vi "Read Trace.vi"(6 "time_bucket":T1(ring), 7 "max points (-1 = all)":i32=-1 min=-1, 8 "error in (no error)":errorcluster, 9 "time interval":T2, 10 "PG path":string, 11 "Data.PGQL in":refnum<class "LV-Data.PGSQL.lvclass">) -> (0 "error out":errorcluster, 1 "Column (units)":string, 2 "Trace":cluster{timestamp[], dbl[]}, 3 "Data.PGSQL out":refnum<class "LV-Data.PGSQL.lvclass">, 5 "SQL string":string)   [LabVIEW 2019, in "LV-Data.PGSQL.lvclass"]
uses:
  LV-Data.PGSQL.lvclass
  Typedefs/Errors--enum.ctl
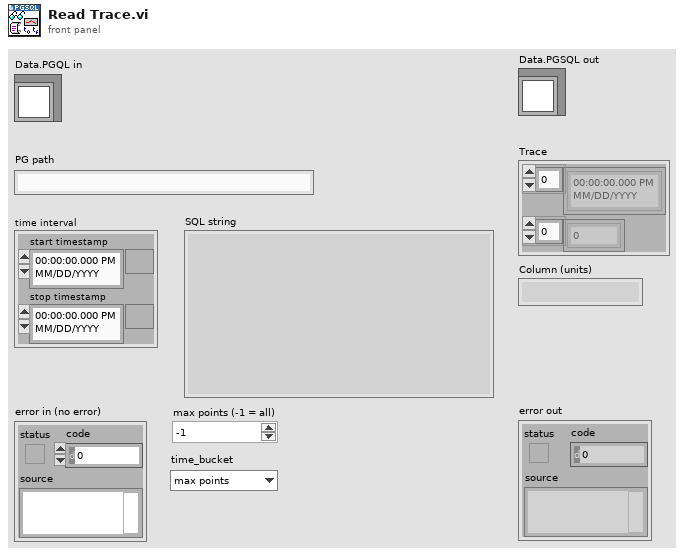
[diagram p1: front panel]
types:
  T1 = enum16{"max points", "1 second", "5 seconds", "10 seconds", "30 seconds", "1 minute", "5 minutes", "10 minutes", "30 minutes", "1 hour", "5 hours", "10 hours", "30 hours"}
  T2 = cluster{"start timestamp":timestamp, "stop timestamp":timestamp}
  T3 = typedef "LV-Data.PGSQL.lvclass/Time.Datatype--enum.ctl" = enum16{"timestamp without time zone", "timestamp with time zone"}
  T4 = typedef "LV-Data.PGSQL.lvclass/Errors--enum.ctl" = enum16{"0: None", "5005: Path Type Not Supported", "5006: Number of Variables", "5007: Number of data points", "5008: Cannot write two data points", "5030: Start and End Times Identical", "5031: Input is not wholly", "5032: Undefined Timestamps", "5033: Bad path or paths", "5040: Invalid Instrument Name", "5050: Column can only hold string", "5051: Column can only hold bool", "5052: Column can only hold double", "5053: Column can only hold int"}
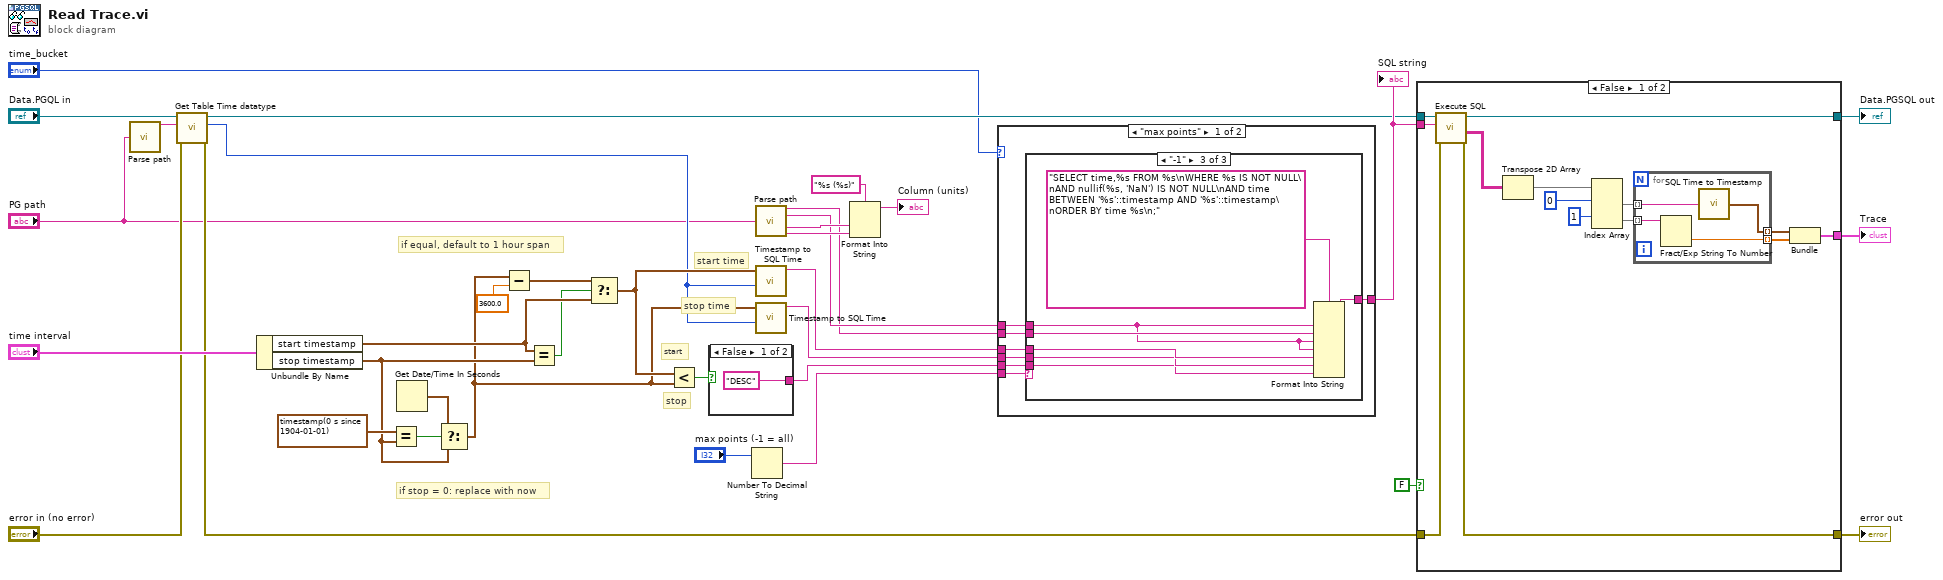
[diagram p0: block diagram]
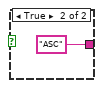
[diagram p2: hidden frame]
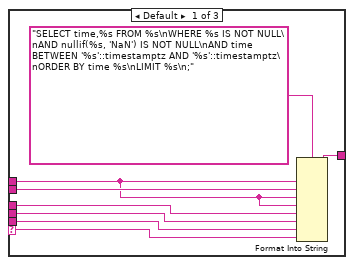
[diagram p3: hidden frame]
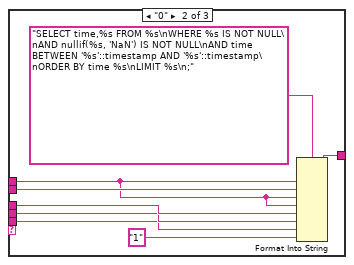
[diagram p4: hidden frame]
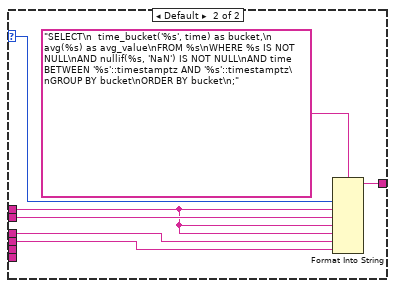
[diagram p5: hidden frame]
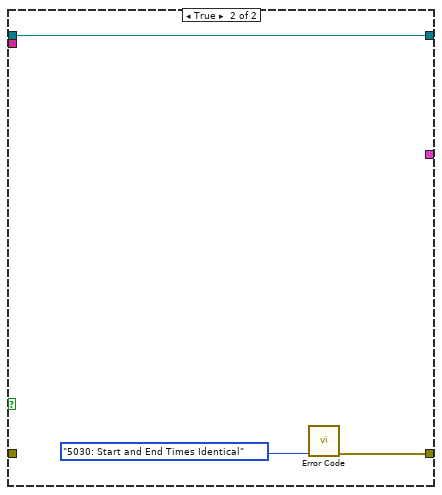
[diagram p6: hidden frame]
diagram:
  # "if equal, default to 1 hour span"
  # "if stop = 0: replace with now"
  # "stop"
  # "start"
  # "stop time"
  # "start time"
  n1 = call "Parse path.vi"("PG Path"="PG path") -> ("Table path"=w7:string)  [unwired: 10 in, 4 out]
  n2 = call "Get Table Time datatype.vi"("error in (no error)"="error in (no error)", "Table path"=w7, "LV-Data.PGSQL in"="Data.PGQL in") -> ("error out"=w5:errorcluster, "Time Datatype"=w3:T3, "LV-Data.PGSQL out"=w4:refnum<class "LV-Data.PGSQL.lvclass">)  [unwired: 6 in]
  n3 = Unbundle By Name("time interval") -> ("start timestamp"=w24:timestamp, "stop timestamp"=w25:timestamp)
  n4 = Equal?(x=timestamp(0 s since 1904-01-01) ("stop timestamp"), y=w25) -> (x = y?=w30:bool)
  n5 = Get Date/Time In Seconds() -> (seconds since 1Jan1904=w27:timestamp)
  n6 = Select(t=w27, s=w30, f=w25) -> (s? t:f=w21:timestamp)
  n7 = Subtract(x=w21, y=3600.0) -> (x-y=w26:timestamp)
  n8 = Equal?(x=w24, y=w25) -> (x = y?=w9:bool)
  n9 = Select(t=w26, s=w9, f=w24) -> (s? t:f=w22:timestamp)
  n10 = Less?(x=w22, y=w21) -> (x < y?=w36:bool)
  n11 = case shown="False" w36 {
    tunnel: ["DESC" "ASC"] -> w12
    frame False {
    }
    frame True {
    }
  }
  n12 = Number To Decimal String(number="max points (-1 = all)") -> (decimal integer string=w11:string)  [unwired: 1 in]
  n13 = call "Parse path.vi"("PG Path"="PG path") -> ("Table path"=w15:string, "Column path"=w16:string, "Column name"=w17:string, "Column units"=w19:string)  [unwired: 10 in, 1 out]
  n14 = call "Timestamp to SQL Time.vi"("Time Datatype"=w3, "Timestamp"=w22) -> ("date/time string"=w14:string)  [unwired: 9 in]
  n15 = call "Timestamp to SQL Time.vi"("Time Datatype"=w3, "Timestamp"=w21) -> ("date/time string"=w13:string)  [unwired: 9 in]
  n16 = Format Into String(format string="%s (%s)", w17, w19) -> (resulting string=→"Column (units)":string)  [unwired: 2 in, 1 out]
  n17 = case shown="\"max points\"" "time_bucket" {
    selector: "time_bucket" -> [_ w74]
    tunnel: w16 -> [w44 w71]
    tunnel: w15 -> [w45 w73]
    tunnel: w14 -> [w43 w69]
    tunnel: w13 -> [w42 w70]
    tunnel: w12 -> [w41 _]
    tunnel: w11 -> [w39 _]
    tunnel: [w40 w72] -> w10
    frame "max points" {
      n18 = case shown="\"-1\"" w39 {
        selector: w39 -> [w47 _ _]
        tunnel: w45 -> [w52 w60 w67]
        tunnel: w44 -> [w46 w54 w62]
        tunnel: w43 -> [w51 w59 w66]
        tunnel: w42 -> [w50 w58 w65]
        tunnel: w41 -> [w49 w57 w64]
        tunnel: [w48 w56 w63] -> w40
        frame Default {
          n19 = Format Into String(format string="SELECT time,%s FROM %s\nWHERE %s IS NOT NULL\nAND nullif(%s, 'NaN') IS NOT NULL\nAND time BETWEEN '%s'::timestamptz AND '%s'::timestamptz\nORDER BY time %s\nLIMIT %s\n;", w46, w52, w46, w46, w51, w50, w49, w47) -> (resulting string=w48:string)  [unwired: 2 in, 1 out]
        }
        frame "0" {
          n20 = Format Into String(format string="SELECT time,%s FROM %s\nWHERE %s IS NOT NULL\nAND nullif(%s, 'NaN') IS NOT NULL\nAND time BETWEEN '%s'::timestamp AND '%s'::timestamp\nORDER BY time %s\nLIMIT %s\n;", w54, w60, w54, w54, w59, w58, w57, "1" ("input 7")) -> (resulting string=w56:string)  [unwired: 2 in, 1 out]
        }
        frame "-1" {
          n21 = Format Into String(format string="SELECT time,%s FROM %s\nWHERE %s IS NOT NULL\nAND nullif(%s, 'NaN') IS NOT NULL\nAND time BETWEEN '%s'::timestamp AND '%s'::timestamp\nORDER BY time %s\n;", w62, w67, w62, w62, w66, w65, w64) -> (resulting string=w63:string)  [unwired: 2 in, 1 out]
        }
      }
    }
    frame Default {
      n22 = Format Into String(format string="SELECT\n  time_bucket('%s', time) as bucket,\n  avg(%s) as avg_value\nFROM %s\nWHERE %s IS NOT NULL\nAND nullif(%s, 'NaN') IS NOT NULL\nAND time BETWEEN '%s'::timestamptz AND '%s'::timestamptz\nGROUP BY bucket\nORDER BY bucket\n;", w74, w71, w73, w71, w71, w69, w70) -> (resulting string=w72:string)  [unwired: 2 in, 1 out]
    }
  }
  "SQL string" <- w10
  n23 = case shown="False" FALSE {
    tunnel: [w82 _] -> w35
    tunnel: w4 -> [w81 w96]
    tunnel: w10 -> [w77 _]
    tunnel: [w79 w94] -> w33
    tunnel: [w78 w96] -> w32
    tunnel: w5 -> [w80 _]
    frame False {
      n24 = call "Execute SQL.vi"("error in"=w80, "SQL"=w77, "LV-Data.PGSQL"=w81) -> ("error out"=w79:errorcluster, "Result"=w76:string[][], "LV-Data.PGSQL out"=w78:refnum<class "LV-Data.PGSQL.lvclass">)  [unwired: 5 in, 1 out]
      n25 = Transpose 2D Array(2D array=w76) -> (transposed array=w89:string[][])
      n26 = Index Array(array=w89, index (row) #1=0 ("index (row)"), index (row) #2=1 ("index (row)")) -> (element #1=w86:string[], element #2=w85:string[])  [unwired: 2 in]
      n27 = for {
        tunnel: w86 -> [w93] mode=indexing
        tunnel: w85 -> [w92] mode=indexing
        tunnel: [w91] -> w83 mode=indexing
        tunnel: [w90] -> w84 mode=indexing
        n28 = Fract/Exp String To Number(string=w92) -> (number=w91:dbl)  [unwired: 3 in, 1 out]
        n29 = call "SQL Time to Timestamp.vi"("date/time string"=w93) -> ("Time Stamp"=w90:timestamp)
      }
      n30 = Bundle(w84, w83) -> (w82:cluster{timestamp[], dbl[]})  [unwired: 1 in]
    }
    frame True {
      n31 = call "Error Code.vi"("Error code"=Errors--enum."5030: Start and End Times Identical") -> ("error out"=w94:errorcluster)  [unwired: 10 in]
    }
  }
  "error out" <- w33
  "Trace" <- w35
  "Data.PGSQL out" <- w32
